vi "Main.vi"(11 "Module Admin":refnum<class "Delacor_lib_QMH_Cloneable Module Admin.lvclass">) -> ()   [LabVIEW 2016, in "MQTT_Client.lvlib"]
doc: "This template is based off of the Queued Message Handler design pattern and the Queued Message Handler project template that ships with LabVIEW.\n\nThe main difference is that the queue is private to this module and communication between modules is performed via Broadcast and Request events.\n\nRequest events are wrapped in public API methods and are handled in the Event Handling Loop (EHL) of this VI. Any module can register for Broadcast events sent by this module. The EHL generates messages based on user interface actions.\n\nThe Message Handling Loop (MHL) processes messages generated by the EHL, or by other messages. The messages are string values, so new messages can be added easily to the Message Cases case structure in the MHL. Each message cluster can also provide an optional value for Message Data, which is a variant that can be converted to whatever message-specific data is required.\n_____\nBased on Delacor QMH Project Template 5.0.0.82."
uses:
  MQTT_Client.lvlib
  <vilib>/Delacor/Delacor QMH/Libraries/Cloneable Module Admin_class/Delacor_lib_QMH_Cloneable Module Admin.lvclass
  C:/Program Files (x86)/National Instruments/LabVIEW 2016/vi.lib/Delacor/Delacor QMH/Libraries/Module Admin_class/Delacor_lib_QMH_Module Admin.lvclass
  <vilib>/LabVIEW Open Source Project/MQTT Client/Client class/Public Events -- cluster.ctl
  <vilib>/LabVIEW Open Source Project/MQTT Control Packets/Control Packets/CONNACK/Connect Return Code -- enum.ctl
  <vilib>/LabVIEW Open Source Project/MQTT Control Packets/Control Packets/PUBLISH/PUBLISH.lvclass
  <vilib>/LabVIEW Open Source Project/MQTT Connection/MQTT_Base/Base Class/Public Events -- cluster.ctl
  Module Data EHL--cluster.ctl
  Module Data MHL--cluster.ctl
  <vilib>/Delacor/Delacor QMH/Libraries/Cloneable Module Admin_class/Delacor_lib_QMH_Cloneable Module Admin.lvclass/Delacor_lib_QMH_Cloneable Module Admin.ctl
  Stop Argument--cluster.ctl
  <vilib>/Delacor/Delacor QMH/Libraries/Message Queue_class/Delacor_lib_QMH_Message Queue.lvclass/Delacor_lib_QMH_Message Queue.ctl
  <vilib>/LabVIEW Open Source Project/MQTT Client/Client class/Client.lvclass
  C:/Program Files (x86)/National Instruments/LabVIEW 2016/vi.lib/LabVIEW Open Source Project/MQTT Connection/MQTT_Base/Base Class/MQTT_Base.lvclass
  <vilib>/LabVIEW Open Source Project/MQTT Control Packets/Control Packets/ControlPacket/QualityOfService -- enum.ctl
  <vilib>/Delacor/Delacor QMH/Libraries/Module Admin_class/Delacor_lib_QMH_Module Admin.lvclass/Delacor_lib_QMH_Module Admin.ctl
  <vilib>/Utility/miscctls.llb/LVPointTypeDef.ctl
  <vilib>/Delacor/Delacor QMH/Libraries/Cloneable Module Admin_class/Delacor_lib_QMH_Get Module ID.vi
  <vilib>/Delacor/Delacor QMH/Libraries/Message Queue_class/Delacor_lib_QMH_Enqueue Message (Single).vi
  <vilib>/Delacor/Delacor QMH/Libraries/Module Admin_class/Delacor_lib_QMH_Get External Launch.vi
  <vilib>/Utility/error.llb/Error Cluster From Error Code.vi
  <vilib>/ErrorRing/Error Ring.xnode
  <vilib>/Delacor/Delacor QMH/Libraries/Message Queue_class/Delacor_lib_QMH_Message Queue.lvclass
  <vilib>/LabVIEW Open Source Project/MQTT Connection/MQTT_Base/Base Class/MQTT_Base.lvclass
  <vilib>/LabVIEW Open Source Project/MQTT Control Packets/Control Packets/CONNACK/CONNACK.lvclass
  <vilib>/LabVIEW Open Source Project/MQTT Control Packets/Control Packets/ControlPacket/ControlPacket.lvclass
panel:
  out "error out":errorcluster
  out "Status":string
  # "This is a DQMH Cloneable Module\nIt can be connected to an MQTT Broker\n1. Go to the virtual Folder called 'MQTT Local Broker'\n2. Run the 'Simple MQTT Broker.vi'\n3. Run The API Tester an Connect to the IP and PORT of the MQTT Broker\n4. Add in the Broker Secction or your Panther Sniffer for DQMH the MQTT Broker\n5. Add a the DQMH Module to the Modules Section of your app\n6. Tap your Module on the app and you'll se all the Status Updated Broadcast\n\n\nPanther Sniffer for DQMH(r) available on \nGoogle Play Store.\nhttps://play.google.com/store/apps/details?id=mx.com.pantherlab.pantherSniffer"
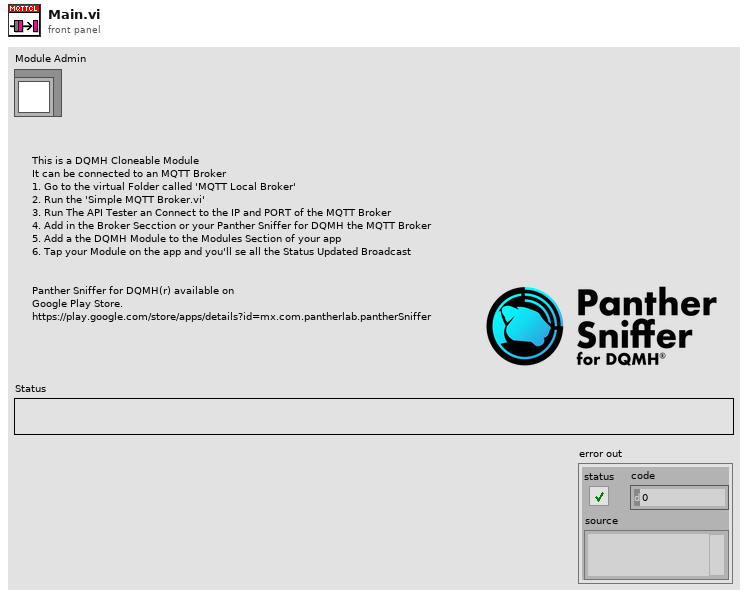
[diagram p1: front panel]
types:
  T1 = typedef "MQTT Base.lvlib/MQTT_Base.lvclass/Public Events -- cluster.ctl" = cluster{"Stop Event":refnum<user-event>, "Error Event":refnum<user-event>, "Inbound Message":refnum<user-event>}
  T2 = typedef "MQTT Client.lvlib/Client.lvclass/Public Events -- cluster.ctl" = cluster{"Connection Status":refnum<user-event>, "Connected":refnum<user-event>, "Application Message":refnum<user-event>}
  T3 = typedef "MQTT_Client.lvlib/Broadcast Events--cluster.ctl" = cluster{"Module Did Init":refnum<user-event>, "Status Updated":refnum<user-event>, "Error Reported":refnum<user-event>, "Module Did Stop":refnum<user-event>, "Update Module Execution Status":refnum<user-event>, "Client Status":refnum<user-event>}
  T4 = typedef "MQTT_Client.lvlib/Request Events--cluster.ctl" = cluster{"Stop Module":refnum<user-event>, "Show Panel":refnum<user-event>, "Hide Panel":refnum<user-event>, "Show Diagram":refnum<user-event>, "Get Module Execution Status":refnum<user-event>, "Connect Client":refnum<user-event>, "Disconnect Client":refnum<user-event>, "Subscribe to topic":refnum<user-event>}
  T5 = typedef "MQTT_Client.lvlib/Module Data MHL--cluster.ctl" = cluster{"Status":string, "Connected":bool}
  T6 = typedef "MQTT_Client.lvlib/Module Data EHL--cluster.ctl" = cluster{"Topics":string[], "Offline?":bool}
  T7 = enum32{"invalid lock state", "Not Locked", "Locked (No Password)", "Password-protected"}
  T8 = typedef "MQTT_Client.lvlib/Stop Argument--cluster.ctl" = cluster{"Module ID":i32, "Origin":string, "Exit via Stop Module Req?":bool, "Wait for Module to stop?":bool}
  T9 = typedef "MQTT_Control_Packets.lvlib/ControlPacket.lvclass/QualityOfService -- enum.ctl" = enum16{"0 (At Most Once)", "1 (At Least Once)", "2 (Exactly Once)"}
  T10 = typedef "LVPointTypeDef.ctl" = cluster{"Horizontal":i16, "Vertical":i16}
  T11 = enum32{"Invalid", "Standard", "Closed", "Hidden", "Minimized", "Maximized"}
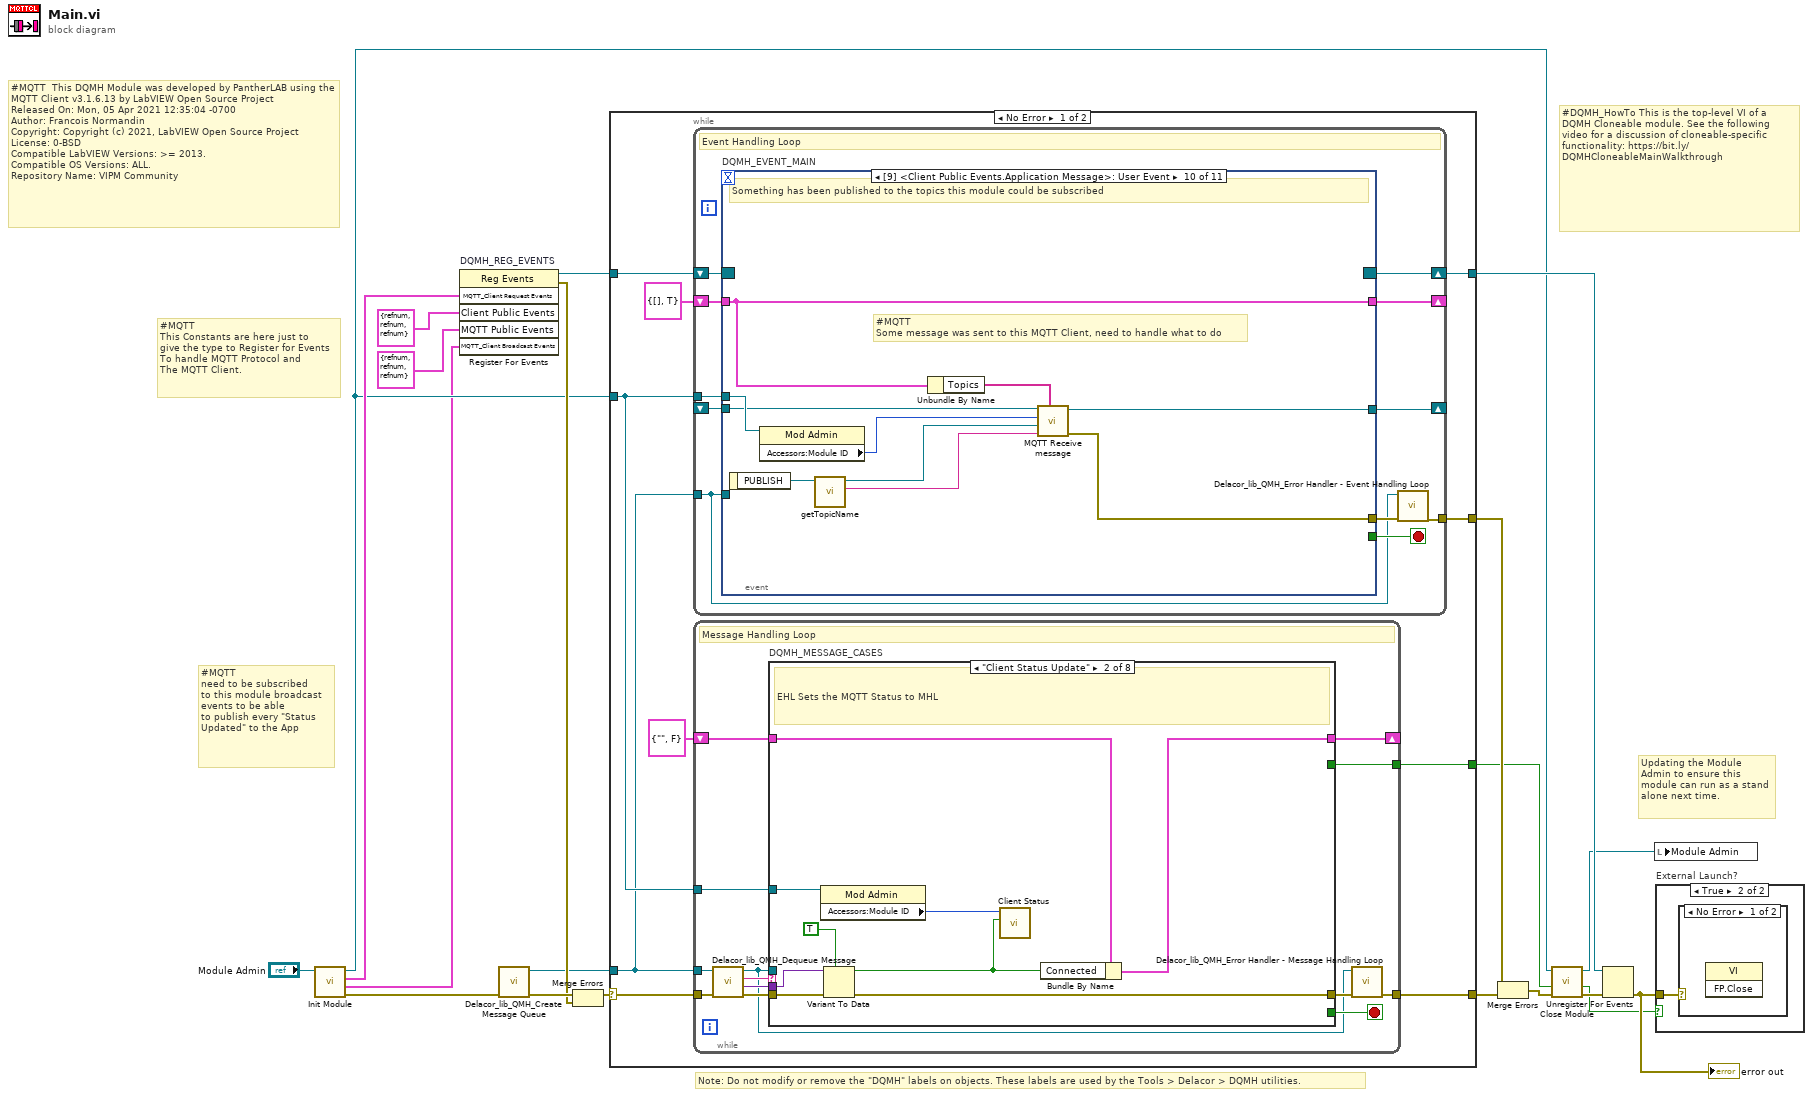
[diagram p0: block diagram]
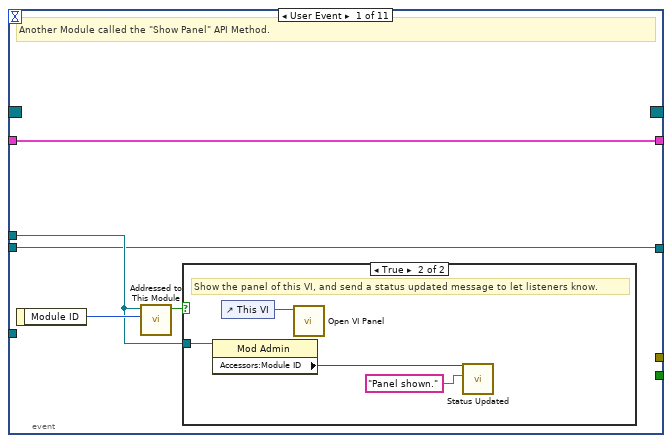
[diagram p2: hidden frame]
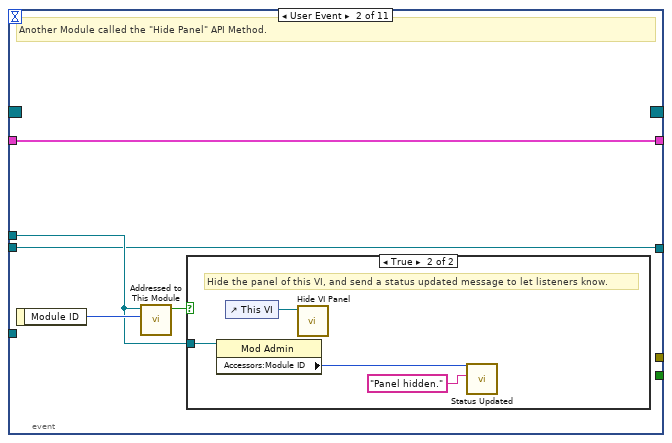
[diagram p4: hidden frame]
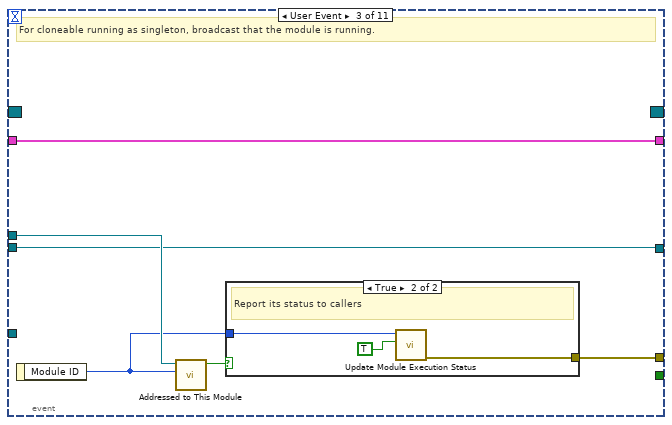
[diagram p6: hidden frame]
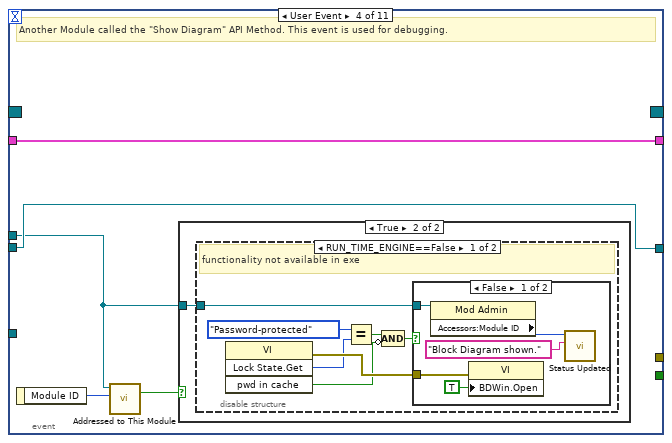
[diagram p8: hidden frame]
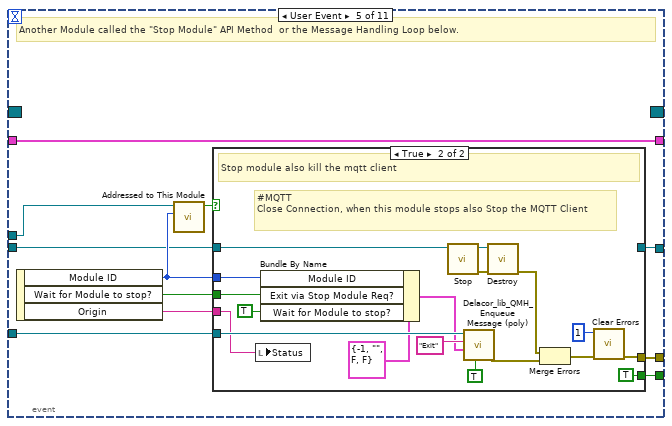
[diagram p12: hidden frame]
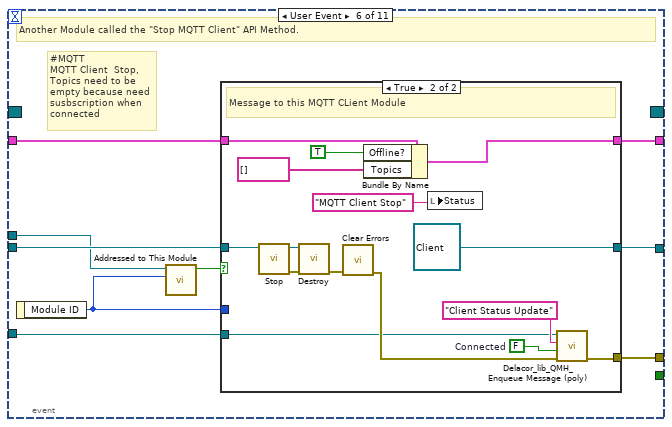
[diagram p14: hidden frame]
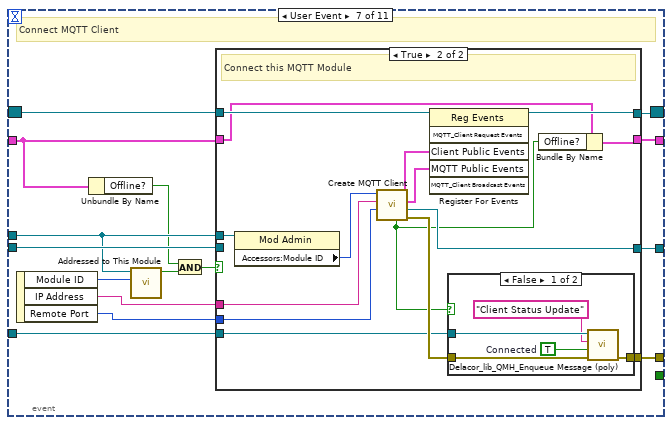
[diagram p16: hidden frame]
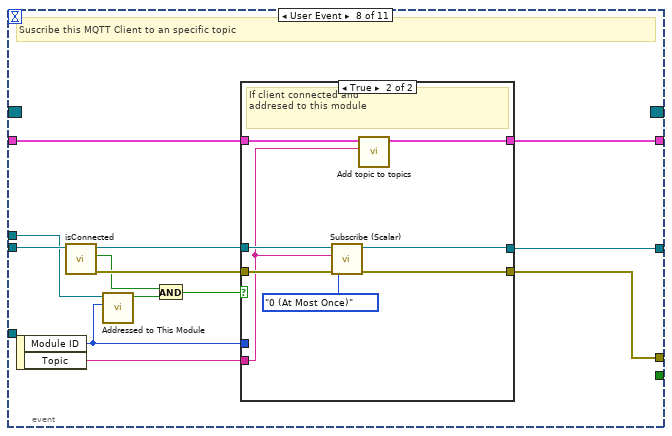
[diagram p19: hidden frame]
diagram:
  # "#MQTT  This DQMH Module was developed by PantherLAB using the \nMQTT Client v3.1.6.13 by LabVIEW Open Source Project\nReleased On: Mon, 05 Apr 2021 12:35:04 -0700\nAuthor: Francois Normandin\nCopyright: Copyright (c) 2021, LabVIEW Open Source Project\nLicense: 0-BSD\nCompatible LabVIEW Versions: >= 2013.\nCompatible OS Versions: ALL.\nRepository Name: VIPM Community"
  # "#MQTT   \nThis Constants are here just to \ngive the type to Register for Events\nTo handle MQTT Protocol and\nThe MQTT Client."
  # "#MQTT   \nneed to be subscribed\nto this module broadcast\nevents to be able\nto publish every \"Status\nUpdated\" to the App"
  # "#DQMH_HowTo This is the top-level VI of a DQMH Cloneable module. See the following video for a discussion of cloneable-specific functionality: https://bit.ly/DQMHCloneableMainWalkthrough"
  # "Note: Do not modify or remove the \"DQMH\" labels on objects. These labels are used by the Tools > Delacor > DQMH utilities."
  # "Updating the Module Admin to ensure this module can run as a stand alone next time."
  n1 = call "Init Module.vi"("Cloneable Module Admin in"="Module Admin") -> ("error out"=w18:errorcluster, "MQTT_Client Broadcast Events"=w1:T3, "MQTT_Client Request Events"=w5:T4, "Cloneable Module Admin out"=w4:refnum<class "Delacor_lib_QMH_Cloneable Module Admin.lvclass">)  [unwired: 7 in]
  n2 = register-events "DQMH_REG_EVENTS"(w5, T2 {"Connection Status"=refnum, "Connected"=refnum, "Application Message"=refnum} ("Client Public Events"), T1 {"Stop Event"=refnum, "Error Event"=refnum, "Inbound Message"=refnum} ("MQTT Public Events"), w1) -> (reference out=w11:refnum<event-registration>, error out=w14:errorcluster)  [unwired: 2 in]
  n3 = call <vilib>:"Delacor_lib_QMH_Create Message Queue.vi"("error in"=w18) -> ("error out"=w16:errorcluster, "Message Queue"=w10:refnum<class "Delacor_lib_QMH_Message Queue.lvclass">)  [unwired: 9 in]
  n4 = Merge Errors(w16, w14) -> (w15:errorcluster)
  n5 = case shown="No Error" w15 {
    selector: w15 -> [w29 w357]
    tunnel: [w31 w356] -> w19
    tunnel: [w28 w355] -> w12
    tunnel: w11 -> [w27 w355]
    tunnel: w10 -> [w24 w348]
    tunnel: [w30 _] -> w20
    tunnel: w4 -> [w26 w351]
    tunnel: [w25 _] -> w7
    frame No Error {
      n6 = while {
        tunnel: w24 -> [w36]
        shift-right: [w39] -> w28
        shift-left: w27 -> [w40]
        tunnel: [w41] -> w30
        tunnel: w26 -> [w37]
        shift-right: [w34] -> _
        shift-left: _ -> [w33]
        shift-right: [w32] -> _
        shift-left: T6 {"Topics"=[], "Offline?"=TRUE} ("Data Cluster") -> [w35]
        stop <- w38 stop-if-true
        # "Event Handling Loop"
        n7 = event "DQMH_EVENT_MAIN" shown="[9] <Client Public Events.Application Message>: User Event" {
          selector: w40 -> [_ _ _ _ _ _ w152 _ _ _ _]
          dyn-events: [_ _ _ _ _ _ w153 _ _ _ _] -> w39
          timeout: _ -> [_ _ _ _ _ _ _ _ _ _ _]
          tunnel: [_ _ _ _ w94 _ _ _ _ _ _] -> w38
          tunnel: w36 -> [_ _ _ _ w97 w118 w144 _ w210 _ _]
          tunnel: [_ _ w66 _ w98 w126 w158 w194 w213 w228 w237] -> w42
          tunnel: w37 -> [w45 w54 w64 w70 w96 w122 w150 w187 w211 w226 w231]
          tunnel: w35 -> [w44 w52 w61 w71 w89 w120 w149 w185 w207 w227 w236]
          tunnel: [w43 w53 w62 w72 w88 w124 w157 w193 w208 w224 w233] -> w34
          tunnel: w33 -> [w43 w53 w62 w72 w90 w123 w155 w190 w208 w223 w234]
          tunnel: [w44 w52 w61 w71 w89 w119 w151 w184 w207 w227 w236] -> w32
          event User Event {
            # "Another Module called the \"Show Panel\" API Method."
            n8 = event-data() -> ("Module ID"=w46:i32)  [unwired: 1 in]
            n9 = call "Addressed to This Module.vi"("Module ID from Argument"=w46, "Module Admin"=w45) -> ("Addressed to this instance?"=w47:bool)  [unwired: 8 in, 1 out]
            n10 = case shown="True" w47 {
              tunnel: w45 -> [_ w49]
              frame False {
              }
              frame True {
                # "Show the panel of this VI, and send a status updated message to let listeners know."
                n11 = property class="Mod Admin"(reference=w49) -> ("Accessors:Module ID"=w48:i32)  [unwired: 1 in, 2 out]
                n12 = control-ref of="This VI"() -> (w51:refnum<vi>)
                n13 = call "Open VI Panel.vi"("VI"=w51) -> ()  [unwired: 10 in, 1 out]
                n14 = call "Status Updated.vi"("Status"="Panel shown." ("format string"), "Module ID"=w48) -> ()  [unwired: 9 in, 1 out]
              }
            }
          }
          event User Event {
            # "Another Module called the \"Hide Panel\" API Method."
            n15 = event-data() -> ("Module ID"=w55:i32)  [unwired: 1 in]
            n16 = call "Addressed to This Module.vi"("Module ID from Argument"=w55, "Module Admin"=w54) -> ("Addressed to this instance?"=w56:bool)  [unwired: 8 in, 1 out]
            n17 = case shown="True" w56 {
              tunnel: w54 -> [_ w58]
              frame False {
              }
              frame True {
                # "Hide the panel of this VI, and send a status updated message to let listeners know."
                n18 = property class="Mod Admin"(reference=w58) -> ("Accessors:Module ID"=w57:i32)  [unwired: 1 in, 2 out]
                n19 = control-ref of="This VI"() -> (w60:refnum<vi>)
                n20 = call "Hide VI Panel.vi"("VI"=w60) -> ()  [unwired: 10 in, 1 out]
                n21 = call "Status Updated.vi"("Status"="Panel hidden." ("format string"), "Module ID"=w57) -> ()  [unwired: 9 in, 1 out]
              }
            }
          }
          event User Event {
            # "For cloneable running as singleton, broadcast that the module is running."
            n22 = event-data() -> ("Module ID"=w63:i32)  [unwired: 1 in]
            n23 = call "Addressed to This Module.vi"("Module ID from Argument"=w63, "Module Admin"=w64) -> ("Addressed to this instance?"=w65:bool)  [unwired: 8 in, 1 out]
            n24 = case shown="True" w65 {
              tunnel: [_ w69] -> w66
              tunnel: w63 -> [_ w68]
              frame False {
              }
              frame True {
                # "Report its status to callers"
                n25 = call "Update Module Execution Status.vi"("Running?"=TRUE, "Module ID"=w68) -> ("error out"=w69:errorcluster)  [unwired: 9 in]
              }
            }
          }
          event User Event {
            # "Another Module called the \"Show Diagram\" API Method. This event is used for debugging."
            n26 = event-data() -> ("Module ID"=w73:i32)  [unwired: 1 in]
            n27 = call "Addressed to This Module.vi"("Module ID from Argument"=w73, "Module Admin"=w70) -> ("Addressed to this instance?"=w74:bool)  [unwired: 8 in, 1 out]
            n28 = case shown="True" w74 {
              tunnel: w70 -> [_ w75]
              frame False {
              }
              frame True {
                n29 = disable-structure shown="RUN_TIME_ENGINE==False" {
                  disable-tunnel: w75 -> [w76 _]
                  frame condition #0 (active) {
                    # "functionality not available in exe"
                    n30 = invoke class="VI" method="Lock State.Get"() -> (error out=w82:errorcluster, "Get Lock State"=w81:T7, "pwd in cache"=w78:bool)  [unwired: 4 in, 1 out]
                    n31 = Equal?(x=T7."Password-protected", y=w81) -> (x = y?=w79:bool)
                    n32 = Compound Arithmetic op=AND(w79, invert w78) -> (w77:bool)
                    n33 = case shown="False" w77 {
                      tunnel: w82 -> [w87 _]
                      tunnel: w76 -> [w84 _]
                      frame False {
                        n34 = property class="Mod Admin"(reference=w84) -> ("Accessors:Module ID"=w83:i32)  [unwired: 1 in, 2 out]
                        n35 = property class="VI"(error in=w87, "BDWin.Open"=TRUE ("Block Diagram Window:Open")) -> ()  [unwired: 1 in, 2 out]
                        n36 = call "Status Updated.vi"("Status"="Block Diagram shown." ("format string"), "Module ID"=w83) -> ()  [unwired: 9 in, 1 out]
                      }
                      frame True {
                        # "Password-protected VI, and the password is not in the cache. Do not show the diagram."
                      }
                    }
                  }
                  frame condition #1 {
                  }
                }
              }
            }
          }
          event User Event {
            # "Another Module called the \"Stop Module\" API Method  or the Message Handling Loop below."
            n37 = event-data() -> ("Module ID"=w92:i32, "Wait for Module to stop?"=w93:bool, "Origin"=w91:string)  [unwired: 1 in]
            n38 = call "Addressed to This Module.vi"("Module ID from Argument"=w92, "Module Admin"=w96) -> ("Addressed to this instance?"=w95:bool)  [unwired: 8 in, 1 out]
            n39 = case shown="True" w95 {
              tunnel: [_ w116] -> w98
              tunnel: w97 -> [_ w109]
              tunnel: [_ TRUE] -> w94
              tunnel: w93 -> [_ w104]
              tunnel: w92 -> [_ w106]
              tunnel: w91 -> [_ w102]
              tunnel: w90 -> [w99 w100]
              tunnel: [w99 _] -> w88
              frame False {
              }
              frame True {
                # "#MQTT   \nClose Connection, when this module stops also Stop the MQTT Client"
                # "Stop module also kill the mqtt client"
                n40 = local write "Status"(w102) -> ()
                n41 = Bundle By Name(cluster=T8 {"Module ID"=-1, "Origin"="", "Exit via Stop Module Req?"=FALSE, "Wait for Module to stop?"=FALSE} ("Stop Argument"), "Module ID"=w106, "Exit via Stop Module Req?"=TRUE, "Wait for Module to stop?"=w104) -> (w103:T8)
                n42 = call <vilib>:"Stop.vi"("MQTT_Base in"=w100) -> ("error out"=w117:errorcluster, "MQTT_Base out"=w101:refnum<class "Client.lvclass">)  [unwired: 8 in, 1 out]
                n43 = call-poly <vilib>:"Delacor_lib_QMH_Enqueue Message (poly).vi"("Priority Message? (F)"=TRUE, "Message Data"=w103, "Message"="Exit", "Message Queue in"=w109) -> ("error out"=w113:errorcluster)  [unwired: 6 in, 1 out]
                n44 = call <vilib>:"Destroy.vi"("error in (no error)"=w117, "MQTT_Base in"=w101) -> ("error out"=w114:errorcluster)  [unwired: 8 in, 1 out]
                n45 = Merge Errors(w114, w113) -> (w115:errorcluster)
                n46 = call <vilib>:"Clear Errors.vi"("error in (no error)"=w115, "specific error code to clear (0: all)"=1) -> ("error out"=w116:errorcluster)  [unwired: 4 in, 1 out]
              }
            }
          }
          event User Event {
            # "#MQTT   \nMQTT Client  Stop,\nTopics need to be\nempty because need\nsusbscription when \nconnected"
            # "Another Module called the \"Stop MQTT Client\" API Method."
            n47 = event-data() -> ("Module ID"=w121:i32)  [unwired: 1 in]
            n48 = call "Addressed to This Module.vi"("Module ID from Argument"=w121, "Module Admin"=w122) -> ("Addressed to this instance?"=w125:bool)  [unwired: 8 in, 1 out]
            n49 = case shown="True" w125 {
              tunnel: w123 -> [w128 w139]
              tunnel: [w128 refnum<class "Client.lvclass"> refnum ("MQTT_Base out")] -> w124
              tunnel: [_ w142] -> w126
              tunnel: w121 -> [_ _]
              tunnel: w120 -> [w127 w135]
              tunnel: [w127 w134] -> w119
              tunnel: w118 -> [_ w129]
              frame False {
                # "Not for this module"
              }
              frame True {
                w130 = FALSE  # Connected
                # "Message to this MQTT CLient Module"
                n50 = call <vilib>:"Stop.vi"("MQTT_Base in"=w139) -> ("error out"=w143:errorcluster, "MQTT_Base out"=w138:refnum<class "Client.lvclass">)  [unwired: 8 in, 1 out]
                n51 = call <vilib>:"Destroy.vi"("error in (no error)"=w143, "MQTT_Base in"=w138) -> ("error out"=w141:errorcluster)  [unwired: 8 in, 1 out]
                n52 = call <vilib>:"Clear Errors.vi"("error in (no error)"=w141) -> ("error out"=w140:errorcluster)  [unwired: 5 in, 1 out]
                n53 = Bundle By Name(cluster=w135, "Offline?"=TRUE ("New Client"), "Topics"=string[] []) -> (w134:T6)
                n54 = local write "Status"("MQTT Client Stop" ("Status")) -> ()
                n55 = call-poly <vilib>:"Delacor_lib_QMH_Enqueue Message (poly).vi"("error in"=w140, "Message Data"=w130, "Message"="Client Status Update", "Message Queue in"=w129) -> ("error out"=w142:errorcluster)  [unwired: 6 in, 1 out]
              }
            }
          }
          event User Event {
            # "Connect MQTT Client"
            n56 = event-data() -> ("Module ID"=w154:i32, "IP Address"=w146:string, "Remote Port"=w145:u16)  [unwired: 1 in]
            n57 = Unbundle By Name(w149) -> ("Offline?"=w147:bool)
            n58 = call "Addressed to This Module.vi"("Module ID from Argument"=w154, "Module Admin"=w150) -> ("Addressed to this instance?"=w156:bool)  [unwired: 8 in, 1 out]
            n59 = And(x=w147, y=w156) -> (x .and. y?=w148:bool)
            n60 = case shown="True" w148 {
              tunnel: [w161 w174] -> w157
              tunnel: w155 -> [w161 _]
              tunnel: [_ w175] -> w158
              tunnel: [w160 w170] -> w153
              tunnel: w152 -> [w160 w173]
              tunnel: w149 -> [w159 w165]
              tunnel: [w159 w164] -> w151
              tunnel: w150 -> [_ w169]
              tunnel: w146 -> [_ w167]
              tunnel: w145 -> [_ w166]
              tunnel: w144 -> [_ w163]
              frame False {
                # "not for this MQTT Client"
              }
              frame True {
                # "Connect this MQTT Module"
                n61 = property class="Mod Admin"(reference=w169) -> ("Accessors:Module ID"=w168:i32)  [unwired: 1 in, 2 out]
                n62 = call "Create MQTT Client.vi"("Remote Port"=w166, "IP Address"=w167, "Module ID"=w168) -> ("error out"=w176:errorcluster, "Client out"=w174:refnum<class "Client.lvclass">, "MQTT Public Events"=w172:T1, "Client Public Events"=w171:T2, "Error connecting?"=w162:bool)  [unwired: 4 in]
                n63 = register-events(reference=w173, w171, w172) -> (reference out=w170:refnum<event-registration>)  [unwired: 3 in, 1 out]
                n64 = case shown="False" w162 {
                  tunnel: w176 -> [w181 w182]
                  tunnel: [w180 w182] -> w175
                  tunnel: w163 -> [w179 _]
                  frame False {
                    w177 = TRUE  # Connected
                    n65 = call-poly <vilib>:"Delacor_lib_QMH_Enqueue Message (poly).vi"("error in"=w181, "Message Data"=w177, "Message"="Client Status Update", "Message Queue in"=w179) -> ("error out"=w180:errorcluster)  [unwired: 6 in, 1 out]
                  }
                  frame True {
                  }
                }
                n66 = Bundle By Name(cluster=w165, "Offline?"=w162) -> (w164:T6)
              }
            }
          }
          event User Event {
            # "Suscribe this MQTT Client to an specific topic"
            n67 = event-data() -> ("Module ID"=w183:i32, "Topic"=w186:string)  [unwired: 1 in]
            n68 = call <vilib>:"isConnected.vi"("Client in"=w190) -> ("error out"=w195:errorcluster, "connected"=w191:bool, "Client out"=w189:refnum<class "Client.lvclass">)  [unwired: 8 in]
            n69 = call "Addressed to This Module.vi"("Module ID from Argument"=w183, "Module Admin"=w187) -> ("Addressed to this instance?"=w192:bool)  [unwired: 8 in, 1 out]
            n70 = And(x=w191, y=w192) -> (x .and. y?=w188:bool)
            n71 = case shown="True" w188 {
              tunnel: w186 -> [_ w202]
              tunnel: w185 -> [w197 w200]
              tunnel: [w197 w199] -> w184
              tunnel: w189 -> [w196 w204]
              tunnel: [w196 w203] -> w193
              tunnel: w195 -> [w198 w206]
              tunnel: [w198 w205] -> w194
              tunnel: w183 -> [_ _]
              frame False {
                # "#MQTT   \nNeeds to be connected to\none MQTT broker and needs\nto be addresed to this module\nthe subscription request"
                # "Not conected or not for this MQTT   Client"
              }
              frame True {
                # "If client connected and\naddresed to this module"
                n72 = call <vilib>:"Subscribe (Scalar).vi"("error in (no error)"=w206, "QoS"=QualityOfService_--_enum."0 (At Most Once)", "Topic Filter"=w202, "Client in"=w204) -> ("error out"=w205:errorcluster, "Client out"=w203:refnum<class "Client.lvclass">)  [unwired: 5 in, 1 out]
                n73 = call "Add topic to topics.vi"("Topic"=w202, "EHL DATA in"=w200) -> ("EHL DATA out"=w199:T6)  [unwired: 9 in]
              }
            }
          }
          event Panel Close? {
            w212 = TRUE  # Discard the event, the MHL is responsible for closing and stopping this VI.
            # "Hide the panel or send the 'Exit' message if the user clicks the 'X' on the module main VI panel."
            n74 = event-data() -> ()  [unwired: 1 in, 1 out]
            n75 = property class="Mod Admin"(reference=w211) -> ("Accessors:External Launch"=w209:bool)  [unwired: 1 in, 2 out]
            n76 = case shown="True" w209 {
              tunnel: w210 -> [_ w217]
              tunnel: [_ w218] -> w213
              frame True {
                # "If externally launched, clicking the 'X' hides the panel, but doesn't close it."
                n77 = control-ref of="This VI"() -> (w214:refnum<vi>)
                n78 = call "Hide VI Panel.vi"("VI"=w214) -> ()  [unwired: 10 in, 1 out]
              }
              frame False {
                # "If run as a stand-alone VI, clicking the panel 'X' stops the VI."
                n79 = call-poly <vilib>:"Delacor_lib_QMH_Enqueue Message (poly).vi"("Priority Message? (F)"=TRUE, "Message"="Exit", "Message Queue in"=w217) -> ("error out"=w218:errorcluster)  [unwired: 7 in, 1 out]
              }
            }
            n80 = event-data("Discard?"=w212) -> ()  [unwired: 1 in, 1 out]
          }
          event User Event {
            # "#MQTT   \nSome message was sent to this MQTT Client, need to handle what to do"
            # "Something has been published to the topics this module could be subscribed"
            n81 = event-data() -> ("PUBLISH"=w225:refnum<class "PUBLISH.lvclass">)  [unwired: 1 in]
            n82 = property class="Mod Admin"(reference=w226) -> ("Accessors:Module ID"=w221:i32)  [unwired: 1 in, 2 out]
            n83 = call <vilib>:"getTopicName.vi"("PUBLISH in"=w225) -> ("Topic"=w219:string, "PUBLISH out"=w220:refnum<class "PUBLISH.lvclass">)  [unwired: 8 in, 1 out]
            n84 = Unbundle By Name(w227) -> ("Topics"=w222:string[])
            n85 = call "MQTT Receive message.vi"("Topics"=w222, "Topic"=w219, "PUBLISH in"=w220, "Accessors:Module ID"=w221, "Client in"=w223) -> ("error out"=w228:errorcluster, "Client out"=w224:refnum<class "Client.lvclass">)  [unwired: 5 in]
          }
          event User Event {
            # "Update Status on the MQTT Topics to be listened by subscribers"
            n86 = event-data() -> ("Module ID"=w230:i32, "Status"=w232:string)  [unwired: 1 in]
            n87 = property class="Mod Admin"(reference=w231) -> ("Accessors:Module ID"=w235:i32)  [unwired: 1 in, 2 out]
            n88 = call "Addressed to This Module.vi"("Module ID from Argument"=w230, "Module Admin"=w231) -> ("Addressed to this instance?"=w229:bool)  [unwired: 8 in, 1 out]
            n89 = case shown="True" w229 {
              tunnel: w235 -> [_ w247]
              tunnel: w234 -> [w238 w246]
              tunnel: [w238 w245] -> w233
              tunnel: [_ w248] -> w237
              tunnel: w232 -> [_ w241]
              frame False {
              }
              frame True {
                # "#MQTT   \n\nThis Module has some status Updated"
                n90 = call "Status updated--constant.vi"() -> ("Topic"=w239:string[])  [unwired: 11 in]
                n91 = call "Format Client MQTT Topics.vi"("Topics Strings"=w239, "Module ID"=w247) -> ("Topics"=w243:string[])  [unwired: 9 in]
                n92 = Index Array(array=w243, index=1) -> (element=w242:string)
                n93 = call <vilib>:"Publish.vi"("QoS"=QualityOfService_--_enum."0 (At Most Once)", "Payload"=w241, "Topic Name (empty: Payload name)"=w242, "Client in"=w246) -> ("error out"=w248:errorcluster, "Client out"=w245:refnum<class "Client.lvclass">)  [unwired: 5 in, 1 out]
              }
            }
          }
        }
        n94 = call-dynamic "Delacor_lib_QMH_Error Handler - Event Handling Loop.vi"("error in"=w42, "Message Queue in"=w36) -> ("dup error in"=w41:errorcluster)  [unwired: 8 in, 1 out]
      }
      n95 = while {
        tunnel: w24 -> [w254]
        tunnel: w29 -> [w260]
        tunnel: [w258] -> w31
        tunnel: w26 -> [w252]
        tunnel: [w251] -> w25
        shift-right: [w249] -> _
        shift-left: T5 {"Status"="", "Connected"=FALSE} ("Module Data") -> [w250]
        stop <- w257 stop-if-true
        # "Message Handling Loop"
        n96 = call-dynamic "Delacor_lib_QMH_Dequeue Message.vi"("error in"=w260, "Message Queue in"=w254) -> ("error out"=w259:errorcluster, "Message Data"=w255:variant, "Message"=w256:string, "Message Queue out"=w253:refnum<class "Delacor_lib_QMH_Message Queue.lvclass">)  [unwired: 6 in]
        n97 = case "DQMH_MESSAGE_CASES" shown="\"Client Status Update\"" w256 {
          selector: w256 -> [_ _ _ _ _ _ _ w336]
          tunnel: w253 -> [_ _ _ _ _ w308 w315 _]
          tunnel: w259 -> [w280 w291 w293 w296 w298 w314 w323 w337]
          tunnel: [w278 w290 w293 w295 w298 w311 w322 w338] -> w261
          tunnel: [_ _ _ _ _ w307 _ _] -> w257
          tunnel: w255 -> [_ w288 _ _ _ w305 w318 _]
          tunnel: w252 -> [w267 w285 _ _ _ w301 w317 w334]
          tunnel: [_ _ _ _ _ w303 _ _] -> w251
          tunnel: w250 -> [w264 w289 w292 w294 w297 w299 w320 w332]
          tunnel: [w263 w286 w292 w294 w297 w299 w320 w332] -> w249
          frame "Initialize" {
            w262 = "Initial Message" ("Initial Message")
            # "Initialize - Any operation that needs to be done before the module can receive messages. Synchronize Caller Events.vi will inform Start Module.vi that the module has launched and is ready to receive messages. Module Did Init.vi will broadcast that the module initialized."
            n98 = call "Synchronize Caller Events.vi"("error in (no error)"=w280, "Module Admin"=w267) -> ("error out"=w279:errorcluster, "Module Admin out"=w266:refnum<class "Delacor_lib_QMH_Cloneable Module Admin.lvclass">)  [unwired: 8 in]
            n99 = property class="Mod Admin"(reference=w266) -> ("Accessors:Module ID"=w269:i32, "Accessors:External Launch"=w268:bool)  [unwired: 1 in, 2 out]
            n100 = call "Module Name--constant.vi"("Module ID"=w269) -> ("Module Name"=w275:string)  [unwired: 10 in]
            n101 = property class="VI"("Front Panel.Title"=w275) -> (reference out=w277:refnum<vi>, error out=w282:errorcluster)  [unwired: 2 in]
            n102 = Select(t=T11."Hidden" ("State"), s=w268, f=T11."Standard" ("State")) -> (s? t:f=w272:T11)
            n103 = invoke class="VI" method="FP.Open"(reference=w277, error in=w282, "State"=w272) -> (reference out=w276:refnum<vi>, error out=w281:errorcluster)  [unwired: 2 in, 3 out]
            n104 = call "Module Name--constant.vi"("Module ID"=w269) -> ("Module Name"=w270:string)  [unwired: 10 in]
            n105 = Bundle By Name(cluster=w264, "Status"=w262) -> (w263:T5)
            n106 = invoke class="VI" method="FP.Center"(reference=w276, error in=w281) -> ()  [unwired: 1 in, 3 out]
            n107 = property on="Pane" class="Pane"("Origin"=T10 {"Horizontal"=0, "Vertical"=0}) -> ()  [unwired: 2 in, 2 out]
            n108 = call "Module Did Init.vi"("error in (no error)"=w279, "Initialized?"=TRUE, "Origin"=w270, "Module ID"=w269) -> ("error out"=w278:errorcluster)  [unwired: 7 in]
            "Status" <- w262
          }
          frame "Client Status Update" {
            # "EHL Sets the MQTT Status to MHL"
            n109 = property class="Mod Admin"(reference=w285) -> ("Accessors:Module ID"=w284:i32)  [unwired: 1 in, 2 out]
            n110 = Variant To Data(error in=w291, type=TRUE, Variant=w288) -> (data=w283:bool, error out=w290:errorcluster)
            n111 = call "Client Status.vi"("Connected"=w283, "Module ID"=w284) -> ()  [unwired: 9 in, 1 out]
            n112 = Bundle By Name(cluster=w289, "Connected"=w283) -> (w286:T5)
          }
          frame "--- Module Specific ---" {
            # "Separator -- The following cases handle messages specific to this Module."
          }
          frame "---Copy This Frame---" {
            # "Duplicate this frame when creating new messages.  Change this comment in the duplicated frame to describe this message."
            n113 = Merge Errors(w296) -> (w295:errorcluster)
          }
          frame "--- Exit and Error Handling---" {
            # "Separator - the following cases handle errors and exit messages."
          }
          frame "Exit" {
            w306 = 91  # 91: not all Exit messages will have an argument
            w307 = TRUE  # Stop the VI
            # "Release the message queue reference"
            # "#CodeNeeded - Add any required cleanup code here."
            # "Exit - Exit the application."
            n114 = Variant To Data(error in=w314, type=T8 {"Module ID"=-1, "Origin"="", "Exit via Stop Module Req?"=FALSE, "Wait for Module to stop?"=FALSE} ("Stop Argument"), Variant=w305) -> (data=w302:T8, error out=w309:errorcluster)
            n115 = call <vilib>:"Clear Errors.vi"("error in (no error)"=w309, "specific error code to clear (0: all)"=w306) -> ("error out"=w313:errorcluster)  [unwired: 4 in, 1 out]
            n116 = control-ref of="This VI"() -> (w300:refnum<vi>)
            n117 = call-dynamic "Delacor_lib_QMH_Release Message Queue.vi"("error in"=w313, "Message Queue"=w308) -> ("error out"=w312:errorcluster)  [unwired: 9 in]
            n118 = call "Handle Exit.vi"("Stop Argument"=w302, "Module Admin in"=w301, "VI reference"=w300) -> ("error out"=w310:errorcluster, "Wait for Stop?"=w303:bool)  [unwired: 7 in]
            n119 = Merge Errors(w312, w310) -> (w311:errorcluster)
          }
          frame "Error" {
            # "#CodeRecommended - If you ever change the name of this \"Error\" message, you'll need to update the name in the Check Loop Error.vi as well."
            # "#CodeRecommended - If the module is running in standalone mode (External Launch = FALSE), this code will pop up an error dialog and call the 'Exit' message if an error occurs. Add more fine-grained error handling here."
            # "Error - Check the error message data and respond accordingly. This message is sent by the \"Error Handler\" VIs at the end of each loop in this application."
            n120 = Variant To Data(error in=w323, type=errorcluster {"status"=FALSE, "code"=0, "source"=""} ("error constant"), Variant=w318) -> (data=w321:errorcluster, error out=w325:errorcluster)
            n121 = property class="Mod Admin"(reference=w317) -> ("Accessors:External Launch"=w319:bool, "Accessors:Module ID"=w316:i32)  [unwired: 1 in, 2 out]
            n122 = call "Error Reported.vi"("Error"=w321, "Module ID"=w316) -> ()  [unwired: 9 in, 1 out]
            n123 = case shown="False" w319 {
              tunnel: [w331 _] -> w324
              tunnel: w321 -> [w330 _]
              tunnel: w315 -> [w327 _]
              frame False {
                # "If the module is running standalone, then pop up an error dialog and call the \"Exit\" message."
                n124 = call <vilib>:"Simple Error Handler.vi"("error in (no error)"=w330) -> ()  [unwired: 4 in, 5 out]
                n125 = call-poly <vilib>:"Delacor_lib_QMH_Enqueue Message (poly).vi"("Priority Message? (F)"=TRUE, "Message"="Exit", "Message Queue in"=w327) -> ("error out"=w331:errorcluster)  [unwired: 7 in, 1 out]
              }
              frame True {
                # "If the module was launched externally, calling the Error Reported broadcast VI is the only action performed by the \"Error\" message. The module's caller can then process the error appropriately."
              }
            }
            n126 = Merge Errors(w325, w324) -> (w322:errorcluster)
            n127 = local write "error out"(w322) -> ()
          }
          frame Default {
            # "'Default' case only runs if there is a message that isn't defined in any of the other cases.  Output a programming error."
            n128 = property class="Mod Admin"(reference=w334) -> ("Accessors:Module ID"=w333:i32)  [unwired: 1 in, 2 out]
            n129 = call "Module Name--constant.vi"("Module ID"=w333) -> ("Module Name"=w335:string)  [unwired: 10 in]
            n130 = xnode "Error Ring"("parameter 0"=w336, "parameter 1"=w335) -> ("error out"=w339:errorcluster)
            n131 = Merge Errors(w337, w339) -> (w338:errorcluster)
          }
        }
        n132 = call-dynamic "Delacor_lib_QMH_Error Handler - Message Handling Loop.vi"("error in"=w261, "Message Queue in"=w253) -> ("dup error in"=w258:errorcluster)  [unwired: 8 in, 1 out]
      }
    }
    frame Error {
      n133 = call "Synchronize Caller Events.vi"("Module Admin"=w351) -> ("Module Admin out"=w350:refnum<class "Delacor_lib_QMH_Cloneable Module Admin.lvclass">)  [unwired: 9 in, 1 out]
      n134 = property class="Mod Admin"(reference=w350) -> ("Accessors:Module ID"=w349:i32)  [unwired: 1 in, 2 out]
      n135 = call-dynamic "Delacor_lib_QMH_Release Message Queue.vi"("error in"=w357, "Message Queue"=w348) -> ("error out"=w356:errorcluster)  [unwired: 9 in]
      n136 = call "Module Name--constant.vi"("Module ID"=w349) -> ("Module Name"=w354:string)  [unwired: 10 in]
      n137 = Format Into String(format string="An error occurred during initialization. %s is no longer running.", w354) -> (resulting string=w352:string)  [unwired: 2 in, 1 out]
      n138 = call "Error Reported.vi"("Additional Information"=w352, "Error"=w356, "Module ID"=w349) -> ()  [unwired: 8 in, 1 out]
    }
  }
  n139 = Merge Errors(w20, w19) -> (w21:errorcluster)
  n140 = call "Close Module.vi"("error in"=w21, "Wait for stop?"=w7, "Module Admin in"=w4) -> ("error out"=w17:errorcluster, "External Launch"=w6:bool, "Module Admin out"=w8:refnum<class "Delacor_lib_QMH_Cloneable Module Admin.lvclass">)  [unwired: 6 in]
  n141 = Unregister For Events(event registration refnum=w12, error in=w17) -> (error out=w13:errorcluster)
  "error out" <- w13
  n142 = local write "Module Admin"(w8) -> ()
  n143 = case "External Launch?" shown="True" w6 {
    tunnel: w13 -> [_ w358]
    frame False {
    }
    frame True {
      n144 = case shown="No Error" w358 {
        frame No Error {
          n145 = invoke class="VI" method="FP.Close"() -> ()  [unwired: 3 in, 3 out]
        }
        frame Error {
          n146 = invoke class="VI" method="FP.Open"("Activate"=TRUE ("Activate?")) -> ()  [unwired: 4 in, 5 out]
        }
      }
    }
  }
